vi "ConnectToScannerUnit.vi"(8 "ComPort":i8=5) -> (0 "error out":errorcluster, 1 "return type":i32=2013)   [LabVIEW 2015]
uses:
  ScannerDiagDLL.dll
panel:
  in  "error in (no error)":errorcluster
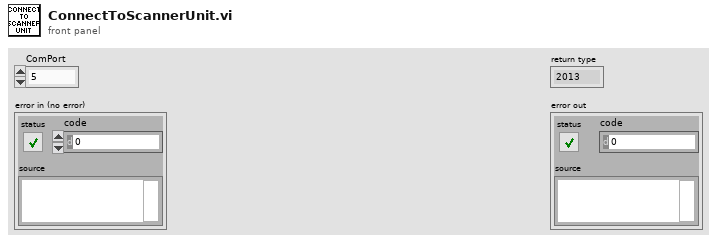
[diagram p1: front panel]
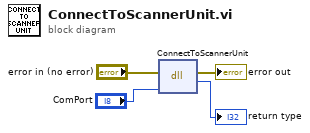
[diagram p0: block diagram]
diagram:
  n1 = dll-call lib="C:/SNAPON/ModisEdge/TabletScope/Test Sequence/Code Modules/DLL/ScannerDiagDLL.dll" fn="ConnectToScannerUnit"(error in="error in (no error)", "ComPort"="ComPort") -> (error out=→"error out":errorcluster, "return type"=→"return type":i32)  [unwired: 3 in, 1 out]
